vi "Get Server Stop UE.vi"(11 "OOP Server in":refnum<class "Streamer_server.lvclass">) -> (2 "Server Stop":refnum<user-event>, 3 "OOP Server out":refnum<class "Streamer_server.lvclass">)   [LabVIEW 2019, in "Streamer_server.lvlib" / "Streamer_server.lvclass"]
uses:
  Streamer_server.lvclass
  Streamer_server.lvclass/Streamer_server.ctl
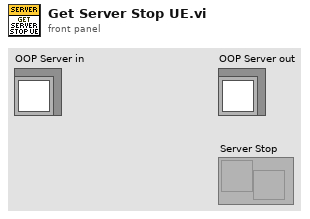
[diagram p1: front panel]
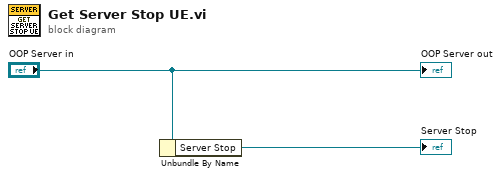
[diagram p0: block diagram]
diagram:
  n1 = Unbundle By Name("OOP Server in") -> ("Server Stop"=→"Server Stop":refnum<user-event>)
  "OOP Server out" <- "OOP Server in"
